vi "setTemp.vi"(11 "Set Temp.":dbl=20.0) -> ()   [LabVIEW 2016]
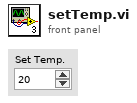
[diagram p1: front panel]
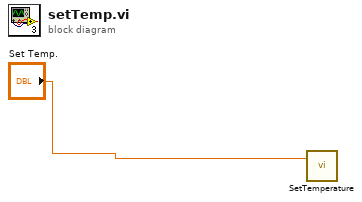
[diagram p0: block diagram]
diagram:
  n1 = call <userlib>:"SetTemperature.vi"("temperature"="Set Temp.") -> ()  [unwired: 1 in, 2 out]
